vi "4Pi Capture Set Interline Interval.vi"(0 "Camera Notifier Name":string, 11 "Frame Rate (Hz)":dbl) -> (4 "Camera Notifier Name (Dup)":string, 15 "Interline Interval (s)":dbl)   [LabVIEW 2021]
uses:
  Device Library/Cameras/Hamamatsu/Orca Flash/Orca Flash Controls/Orca Flash Actions.ctl
  Device Library/Cameras/Hamamatsu/Orca Flash/Orca Flash Controls/Orca Flash Parameters.ctl
  Device Library/Cameras/Hamamatsu/Orca Flash/Orca Flash Controls/Orca Flash Parameter List.ctl
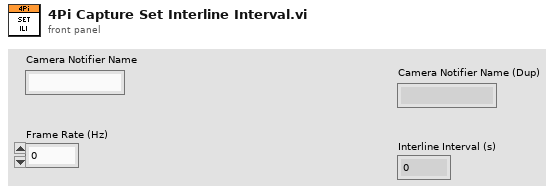
[diagram p1: front panel]
types:
  T1 = typedef "Orca Flash Parameters.ctl" = cluster{"Value":dbl, "Orca Flash Parameters":T2}
  T2 = typedef "Orca Flash Parameter List.ctl" = u32
  T3 = typedef "Orca Flash Actions.ctl" = enum16{"IDLE", "PREVIEW", "RECORD", "Send Trigger", "SOFT TRIGGER", "Record Settings", "SETPARAM", "GETPARAM", "SETROI", "GETROI", "PROGRESSIVE MODE", "AREA MODE", "STATUS", "QUIT"}
  T4 = typedef "Orca Flash ROI.ctl" = cluster{"H Offset":i32, "V Offset":i32, "H Width":i32, "V Width":i32}
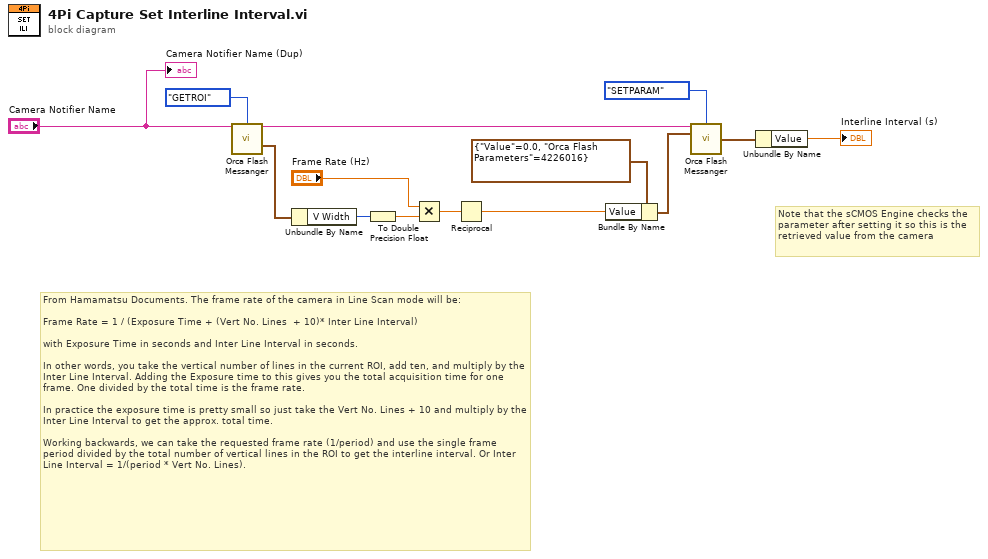
[diagram p0: block diagram]
diagram:
  # "Note that the sCMOS Engine checks the parameter after setting it so this is the retrieved value from the camera"
  # "From Hamamatsu Documents. The frame rate of the camera in Line Scan mode will be:\n\nFrame Rate = 1 / (Exposure Time + (Vert No. Lines  + 10)* Inter Line Interval)\n\nwith Exposure Time in seconds and Inter Line Interval in seconds.\n\nIn other words, you take the vertical number of lines in the current ROI, add ten, and multiply by the Inter Line Interval. Adding the Exposure time to this gives you the total acquisition time for one frame. One divided by the total time is the frame rate.\n\nIn practice the exposure time is pretty small so just take the Vert No. Lines + 10 and multiply by the Inter Line Interval to get the approx. total time.\n\nWorking backwards, we can take the requested frame rate (1/period) and use the single frame period divided by the total number of vertical lines in the ROI to get the interline interval. Or Inter Line Interval = 1/(period * Vert No. Lines)."
  n1 = call "Orca Flash Messanger.vi"("Notifier Name"="Camera Notifier Name", "Camera Actions"=Orca_Flash_Actions."GETROI") -> ("Notifier Name Dup"=w6:string, "sCMOS ROI"=w13:T4)  [unwired: 9 in, 3 out]
  n2 = Unbundle By Name(w13) -> ("V Width"=w12:i32)
  n3 = To Double Precision Float(number=w12) -> (double precision float=w11:dbl)
  n4 = Multiply(x="Frame Rate (Hz)", y=w11) -> (x*y=w9:dbl)
  n5 = Reciprocal(x=w9) -> (1/x=w5:dbl)
  n6 = Bundle By Name(cluster=T1 {"Value"=0.0, "Orca Flash Parameters"=4226016} ("sCMOS Parameter"), "Value"=w5) -> (w4:T1)
  n7 = call "Orca Flash Messanger.vi"("Notifier Name"=w6, "Camera Actions"=Orca_Flash_Actions."SETPARAM", "sCMOS Parameter"=w4) -> ("sCMOS Parameter"=w3:T1)  [unwired: 8 in, 4 out]
  n8 = Unbundle By Name(w3) -> ("Value"=→"Interline Interval (s)":dbl)
  "Camera Notifier Name (Dup)" <- "Camera Notifier Name"
